vi "RDV-sortKeysAlphabeticly.vi"(8 "error in (no error)":errorcluster, 11 "RDV-Reflection_Data_viewer in":refnum<class "RDV-Reflection_Data_viewer.lvclass">) -> (0 "error out":errorcluster, 3 "RDV-Reflection_Data_viewer out":refnum<class "RDV-Reflection_Data_viewer.lvclass">)   [LabVIEW 2020, in "RDV-Reflection_Data_viewer.lvclass"]
uses:
  RDV-Reflection_Data_viewer.lvclass
  RDV-Reflection_Data_viewer.lvclass/RDV-Reflection_Data_viewer.ctl
  1bc6baab-a834-4652-b74b-bc8157ec794b.vi
  <vilib>/Comparison/Less/Less Functor/Less Functor.lvclass
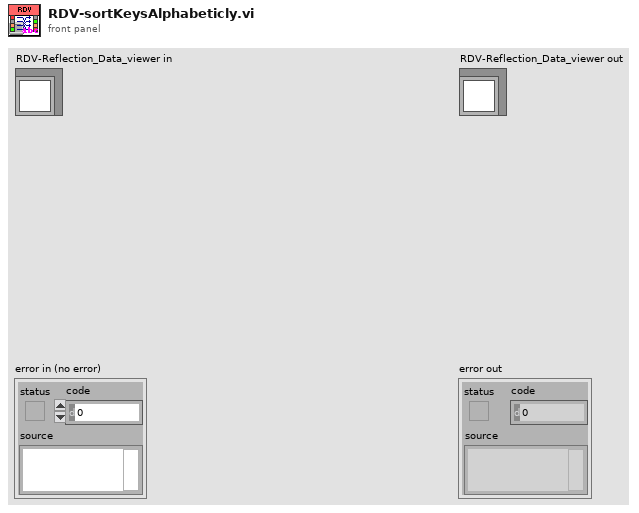
[diagram p1: front panel]
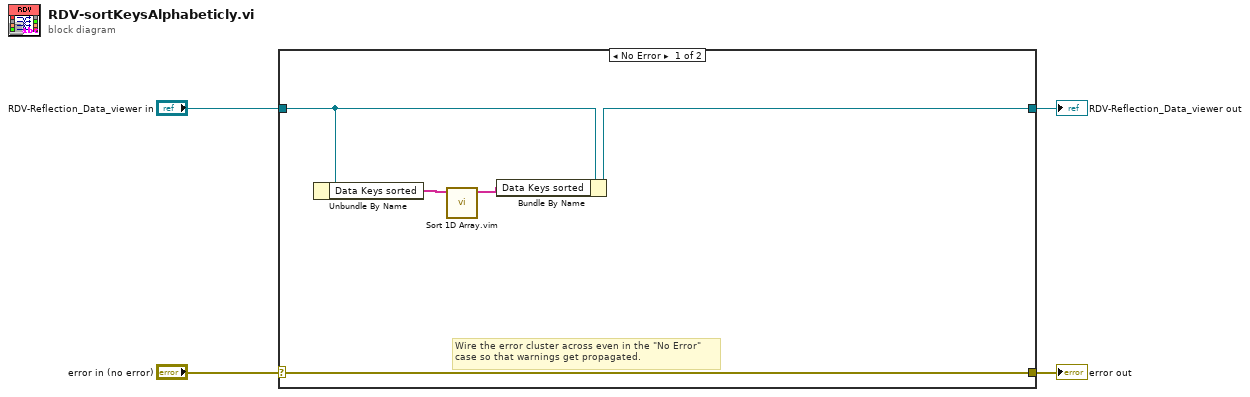
[diagram p0: block diagram]
diagram:
  n1 = case shown="No Error" "error in (no error)" {
    selector: "error in (no error)" -> [w9 w11]
    tunnel: [w9 w11] -> w3
    tunnel: [w5 w10] -> w1
    tunnel: "RDV-Reflection_Data_viewer in" -> [w6 w10]
    frame No Error {
      # "Wire the error cluster across even in the \"No Error\"\ncase so that warnings get propagated."
      n2 = Unbundle By Name(w6) -> ("Data Keys sorted"=w8:string[])
      n3 = call "Sort 1D Array.vim"("unsorted array"=w8) -> ("sorted array"=w7:string[])  [unwired: 10 in]
      n4 = Bundle By Name(cluster=w6, "Data Keys sorted"=w7) -> (w5:refnum<class "RDV-Reflection_Data_viewer.lvclass">)
    }
    frame Error {
    }
  }
  "error out" <- w3
  "RDV-Reflection_Data_viewer out" <- w1
